vi "libssh2_init.vi"(8 "error in (no error)":errorcluster, 11 "path (use built-in)":path) -> (0 "error out":errorcluster, 3 "return value":i32)   [LabVIEW 2013, in "libssh2.lvlib"]
doc: "Initializes libssh2 using the library specified by <B>path</B>."
uses:
  libssh2.lvlib
  Global Settings.vi
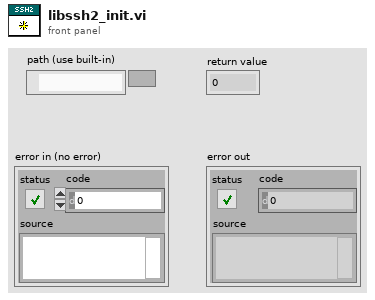
[diagram p1: front panel]
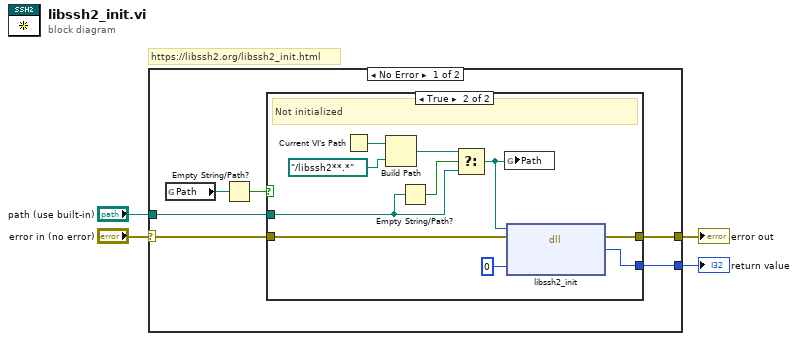
[diagram p0: block diagram]
diagram:
  # "https://libssh2.org/libssh2_init.html"
  n1 = case shown="No Error" "error in (no error)" {
    selector: "error in (no error)" -> [w8 w22]
    tunnel: [w10 _] -> w4
    tunnel: [w9 w22] -> w3
    tunnel: "path (use built-in)" -> [w7 _]
    frame No Error {
      n2 = global read "Global Settings.vi" "Path"() -> (w5:path)
      n3 = Empty String/Path?(string/path=w5) -> (empty?=w6:bool)
      n4 = case shown="True" w6 {
        tunnel: [_ w20] -> w10
        tunnel: [w11 w19] -> w9
        tunnel: w8 -> [w11 w18]
        tunnel: w7 -> [_ w16]
        frame False {
          # "Already initialized"
        }
        frame True {
          # "Not initialized"
          n5 = Current VI's Path() -> (path=w14:path)
          n6 = Build Path(base path=w14, name or relative path=path "../libssh2**.*") -> (appended path=w13:path)
          n7 = Empty String/Path?(string/path=w16) -> (empty?=w17:bool)
          n8 = Select(t=w13, s=w17, f=w16) -> (s? t:f=w15:path)
          n9 = global write "Global Settings.vi" "Path"(w15) -> ()
          n10 = dll-call lib="C:/Users/pasca/source/repos/libssh2-labview/libssh2/libssh2**.*" fn="libssh2_init"(path in=w15, error in=w18, "flags"=0) -> (error out=w19:errorcluster, "return value"=w20:i32)  [unwired: 2 in, 1 out]
        }
      }
    }
    frame Error {
    }
  }
  "error out" <- w3
  "return value" <- w4
